vi "memory leak.vi"() -> ()   [LabVIEW 2024, in "Test Cases.lvclass"]
uses:
  Test Cases.lvclass
  D:/git/Sourcegrid-LabVIEW/dll/SourceGrid.dll
  dll/SourceGrid.dll
  source/Grid/SourceGrid.lvclass
  source/Cells/Check Box/Check Box.lvclass
  D:/git/Sourcegrid-LabVIEW/source/Cells/Cell/Cell.lvclass
  source/Grid/Set Column Default Width.vi
panel:
  in  "Grid Container":refnum<k24>(container)
  in  "stop":bool
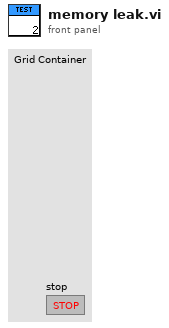
[diagram p1: front panel]
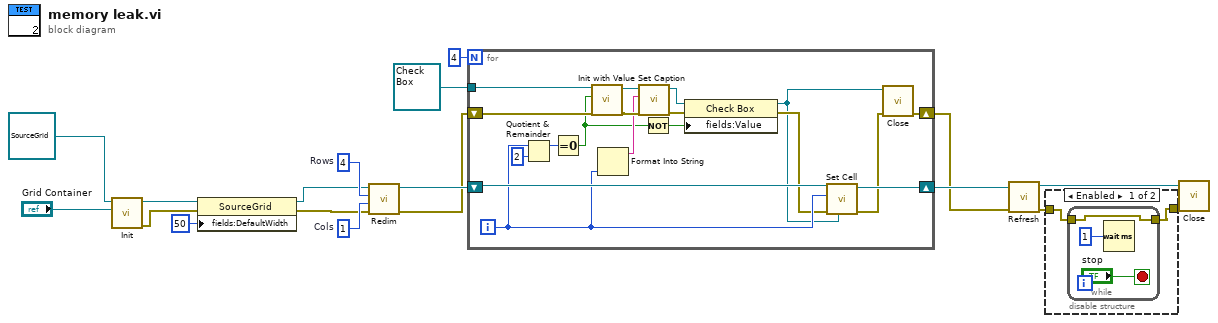
[diagram p0: block diagram]
diagram:
  w17 = 1  # Cols
  w18 = 4  # Rows
  n1 = call-dynamic "Init.vi"("Sourcegrid Container"="Grid Container", "Grid in"=refnum<class "SourceGrid.lvclass"> refnum) -> ("error out"=w6:errorcluster, "Grid out"=w15:refnum<class "SourceGrid.lvclass">)  [unwired: 8 in]
  n2 = property class="SourceGrid"(reference=w15, error in=w6, "fields:DefaultWidth"=50 ("DefaultWidth")) -> (reference out=w14:refnum<class "SourceGrid.lvclass">, error out=w13:errorcluster)
  n3 = call "Redim.vi"("error in"=w13, "Columns"=w17, "Rows"=w18, "Sourcegrid in"=w14) -> ("error out"=w1:errorcluster, "Sourcegrid out"=w10:refnum<class "SourceGrid.lvclass">)  [unwired: 6 in]
  n4 = for {
    N: 4 -> [_]
    shift-right: [w34] -> w2
    shift-left: w1 -> [w31]
    shift-right: [w36] -> w11
    shift-left: w10 -> [w35]
    tunnel: refnum<class "Check Box.lvclass"> refnum ("Cell in") -> [w32]
    i -> [w25]
    n5 = Quotient & Remainder(x=w25, y=2) -> (x-y*floor(x/y)=w28:i32)  [unwired: 1 out]
    n6 = Equal To 0?(x=w28) -> (x = 0?=w21:bool)
    n7 = call-dynamic "Init with Value.vi"("error in"=w31, "Value"=w21, "Check Box in"=w32) -> ("error out"=w30:errorcluster, "Check Box out"=w26:refnum<class "Check Box.lvclass">)  [unwired: 7 in]
    n8 = Format Into String(w25) -> (resulting string=w24:string)  [unwired: 3 in, 1 out]
    n9 = call-dynamic "Set Caption.vi"("error in"=w30, "Caption"=w24, "Check Box in"=w26) -> ("error out"=w27:errorcluster, "Check Box out"=w22:refnum<class "Check Box.lvclass">)  [unwired: 7 in]
    n10 = Not(x=w21) -> (.not. x?=w20:bool)
    n11 = property class="Check Box"(reference=w22, error in=w27, "fields:Value"=w20) -> (reference out=w19:refnum<class "Check Box.lvclass">, error out=w23:errorcluster)
    n12 = call "Set Cell.vi"("Cell"=w19, "error in"=w23, "Row"=w25, "Sourcegrid in"=w35) -> ("error out"=w33:errorcluster, "Sourcegrid out"=w36:refnum<class "SourceGrid.lvclass">)  [unwired: 6 in]
    n13 = call-dynamic "Close.vi"("error in"=w33, "Cell in"=w19) -> ("error out"=w34:errorcluster)  [unwired: 8 in, 1 out]
  }
  n14 = call "Refresh.vi"("error in"=w2, "SourceGrid in"=w11) -> ("error out"=w4:errorcluster, "SourceGrid out"=w8:refnum<class "SourceGrid.lvclass">)  [unwired: 8 in]
  n15 = disable-structure shown="Enabled" {
    disable-tunnel: w4 -> [w38 w42]
    disable-tunnel: [w37 w42] -> w3
    frame Enabled {
      n16 = while {
        tunnel: w38 -> [w39]
        tunnel: [w39] -> w37
        stop <- "stop" stop-if-true
        n17 = Wait (ms)(milliseconds to wait=u32 1) -> ()  [unwired: 1 out]
      }
    }
    frame Disabled {
    }
  }
  n18 = call-dynamic "Close.vi"("error in"=w3, "Sourcegrid in"=w8) -> ()  [unwired: 8 in, 2 out]
